vi "Cluster(Bundle and unbundle).vi"() -> ()   [LabVIEW 2018]
panel:
  out "Boolean 2":bool
  out "String 2":string
  out "Numeric 2":dbl
  in  "Boolean":bool
  in  "String":string
  in  "Numeric":dbl
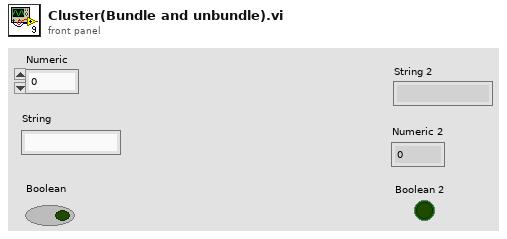
[diagram p1: front panel]
types:
  T1 = cluster{"Numeric":dbl, "String":string, "Boolean":bool}
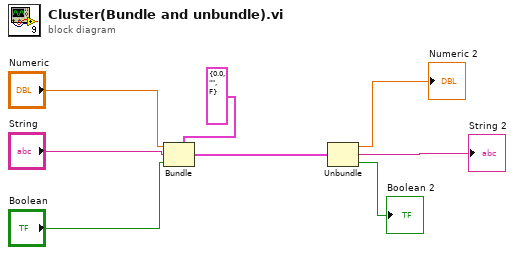
[diagram p0: block diagram]
diagram:
  n1 = Bundle(cluster=T1 {"Numeric"=0.0, "String"="", "Boolean"=FALSE}, "Numeric"="Numeric", "String"="String", "Boolean"="Boolean") -> (w5:T1)
  n2 = Unbundle(w5) -> ("Numeric"=→"Numeric 2":dbl, "String"=→"String 2":string, "Boolean"=→"Boolean 2":bool)
